vi "GetDVRref.vi"(8 "error in (no error)":errorcluster, 11 "Multiply in":refnum<class "Multiply.lvclass">) -> (0 "error out":errorcluster, 2 "data value reference":refnum<data-value>, 3 "Multiply out":refnum<class "Multiply.lvclass">)   [LabVIEW 2023, in "Multiply.lvclass"]
uses:
  Multiply.lvclass
  C:/Users/santharu.subramanian/Documents/LV New Assignments/DVR in OOPS/Classes/Arithmetic/Arithmetic.lvclass
  Arithmetic/Arithmetic.lvclass
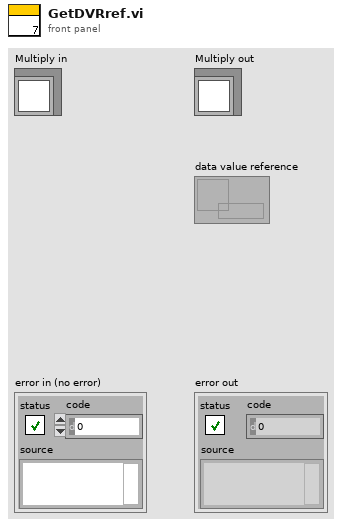
[diagram p1: front panel]
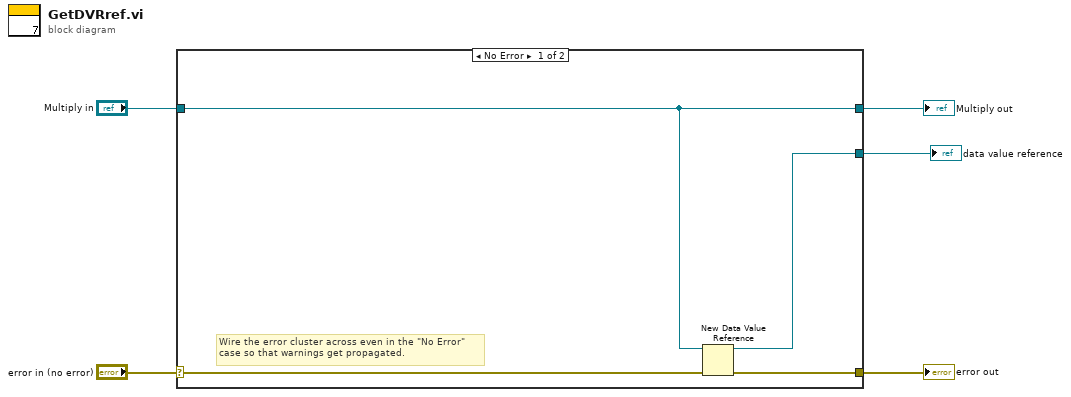
[diagram p0: block diagram]
diagram:
  n1 = case shown="No Error" "error in (no error)" {
    selector: "error in (no error)" -> [w7 w11]
    tunnel: [w6 w11] -> w4
    tunnel: [w8 w10] -> w2
    tunnel: "Multiply in" -> [w8 w10]
    tunnel: [w9 _] -> w1
    frame No Error {
      # "Wire the error cluster across even in the \"No Error\"\ncase so that warnings get propagated."
      n2 = New Data Value Reference(data value=w8, error in=w7) -> (data value reference=w9:refnum<data-value>, error out=w6:errorcluster)
    }
    frame Error {
    }
  }
  "error out" <- w4
  "Multiply out" <- w2
  "data value reference" <- w1
